vi "discount.vi"(8 "member":bool=TRUE, 10 "flavor":string, 11 "size":dbl) -> (2 "discount":dbl)   [LabVIEW 2023]
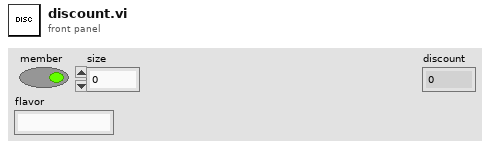
[diagram p1: front panel]
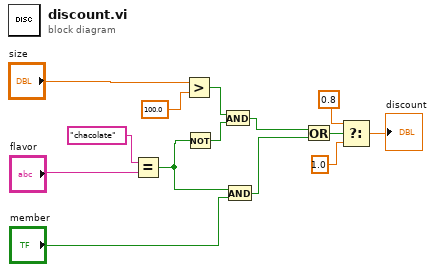
[diagram p0: block diagram]
diagram:
  n1 = Equal?(x="chacolate", y="flavor") -> (x = y?=w5:bool)
  n2 = Greater?(x="size", y=100.0) -> (0:w11:bool)
  n3 = Not(x=w5) -> (.not. x?=w6:bool)
  n4 = And(x=w11, y=w6) -> (x .and. y?=w7:bool)
  n5 = And(x=w5, y="member") -> (x .and. y?=w3:bool)
  n6 = Or(x=w7, y=w3) -> (x .or. y?=w10:bool)
  n7 = Select(t=0.8, s=w10, f=1.0) -> (s? t:f=→"discount":dbl)
